vi "Final GUI.vi"() -> ()   [LabVIEW 2012]
uses:
  <vilib>/Utility/inputDevices.llb/closeJoystick.vi
  <vilib>/Utility/inputDevices.llb/joystickAcquire.vi
panel:
  in  "Request Barometer":bool
  in  "LEDs":bool
  in  "Request temperature":bool
  out "Water in control box?":bool
  out "joystick info":T1(array[cluster])
  out "Temperature (°C)":string
  out "Water Depth (cm)":string
  out "Volt (V)":string
  out "Concatenated string":string
  in  "Joystick index":i32
  in  "Local Port":u16
  out "direction info":T2
  out "button info":T3
  out "axis info":T4
  out "All Data recieved":string
  in  "Remote Port":u16
  in  "Remote Host":string
  in  "stop":bool
  # "All Data"
  # "Setup"
  # "Useless info"
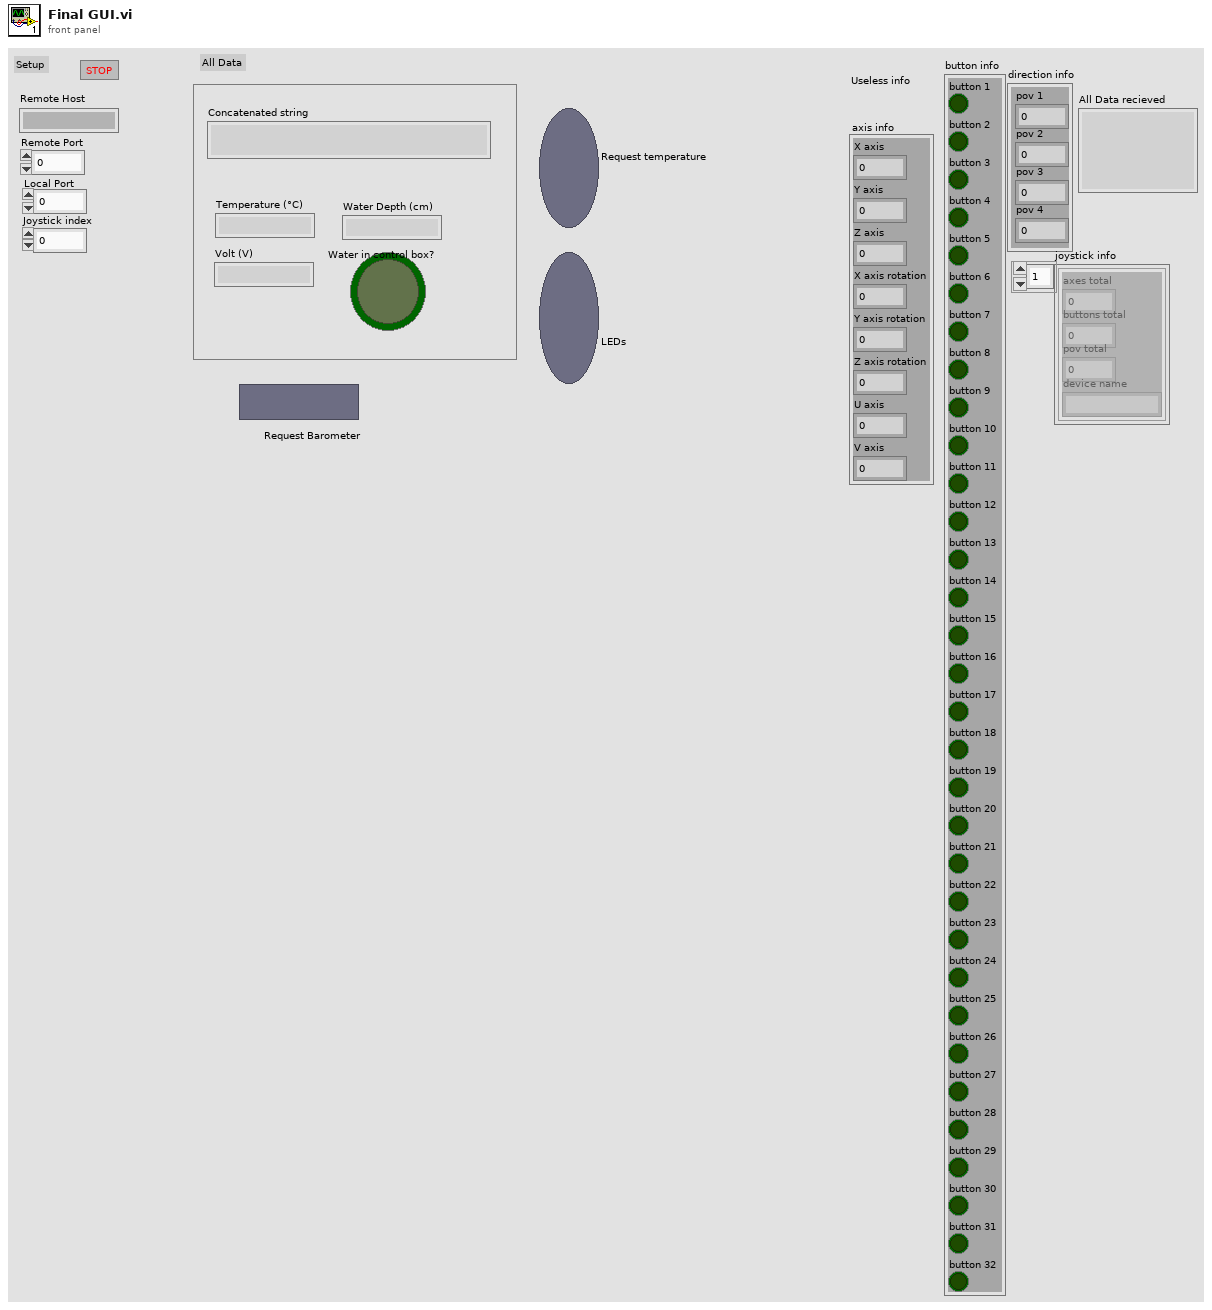
[diagram p1: front panel]
types:
  T1 = cluster{"axes total":u32, "buttons total":u32, "pov total":u32, "device name":string}[]
  T2 = cluster{"pov 1":i32, "pov 2":i32, "pov 3":i32, "pov 4":i32}
  T3 = cluster{"button 1":bool, "button 2":bool, "button 3":bool, "button 4":bool, "button 5":bool, "button 6":bool, "button 7":bool, "button 8":bool, "button 9":bool, "button 10":bool, "button 11":bool, "button 12":bool, "button 13":bool, "button 14":bool, "button 15":bool, "button 16":bool, "button 17":bool, "button 18":bool, "button 19":bool, "button 20":bool, "button 21":bool, "button 22":bool, "button 23":bool, "button 24":bool, "button 25":bool, "button 26":bool, "button 27":bool, "button 28":bool, "button 29":bool, "button 30":bool, "button 31":bool, "button 32":bool}
  T4 = cluster{"X axis":i32, "Y axis":i32, "Z axis":i32, "X axis rotation":i32, "Y axis rotation":i32, "Z axis rotation":i32, "U axis":i32, "V axis":i32}
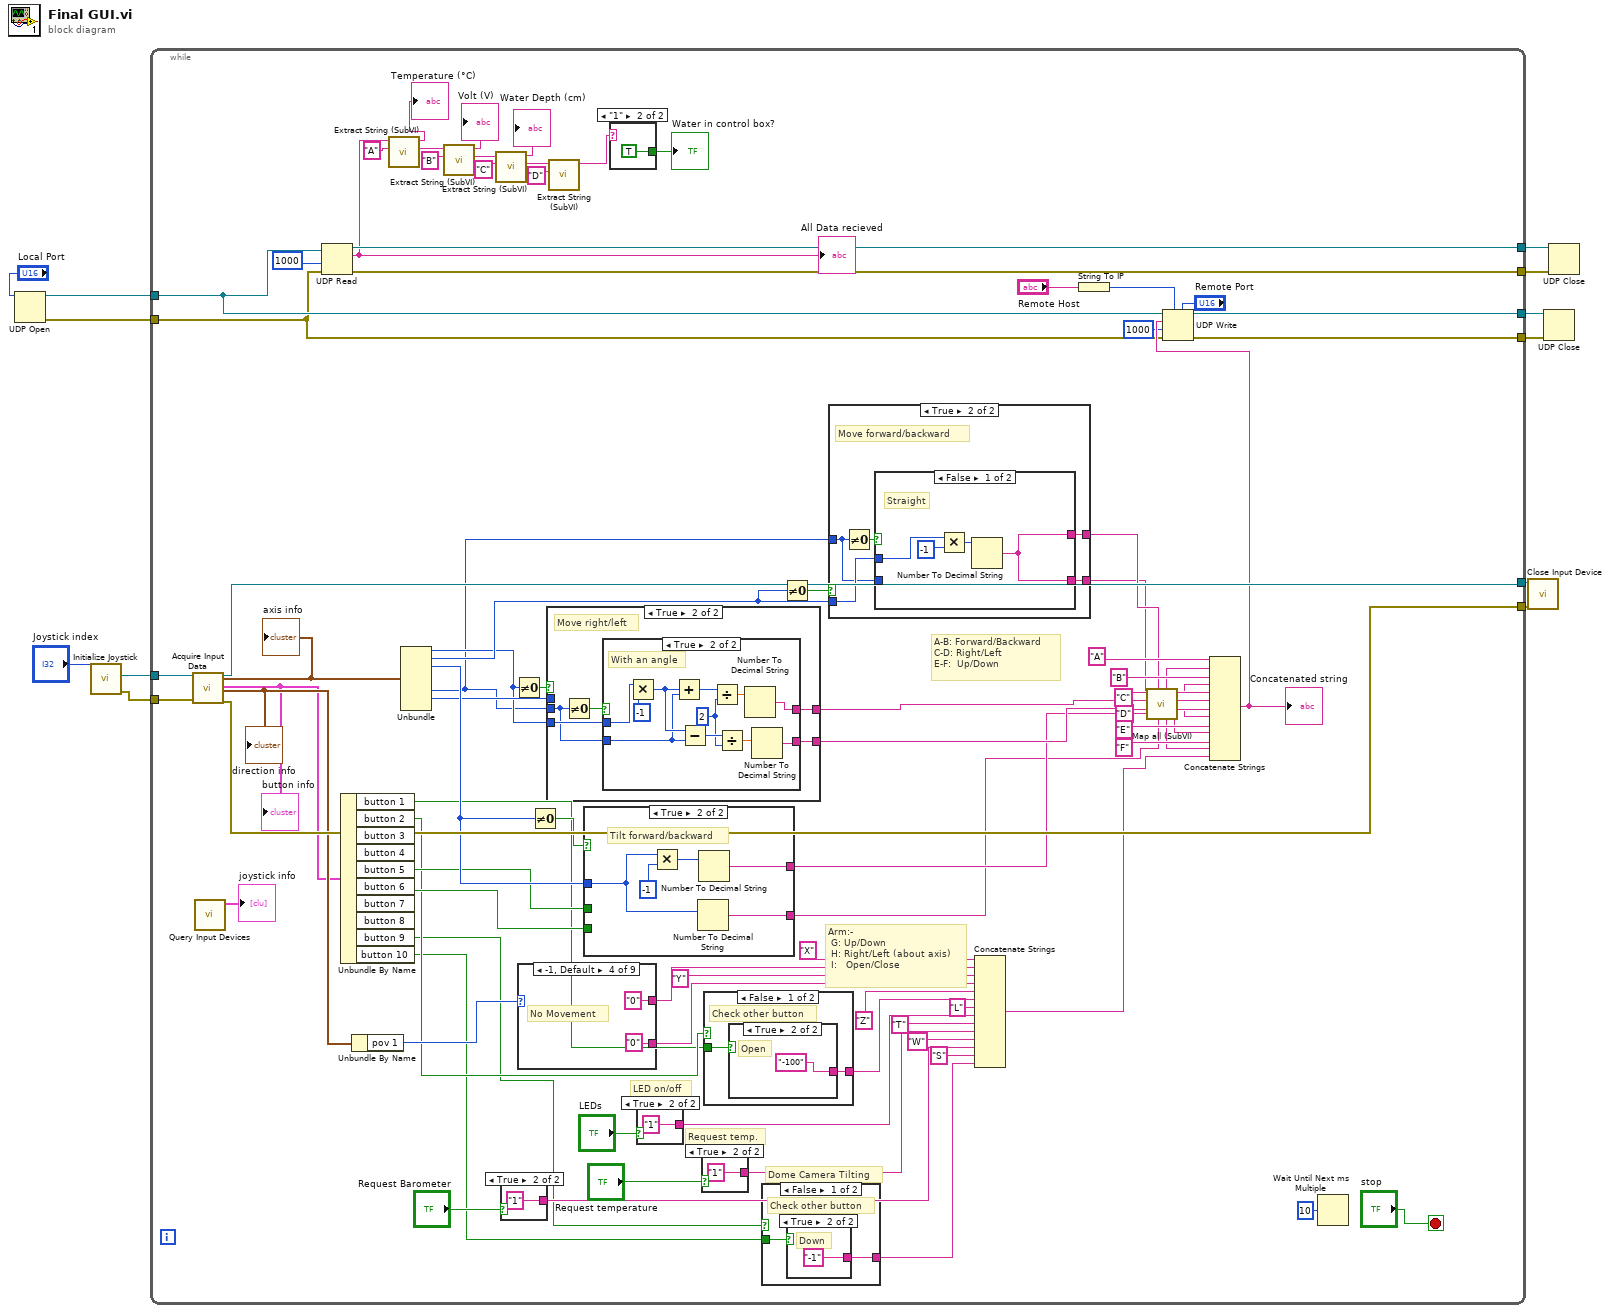
[diagram p0: block diagram]
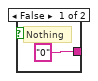
[diagram p2: hidden frame]
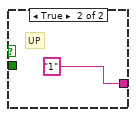
[diagram p3: hidden frame]
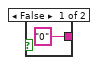
[diagram p4: hidden frame]
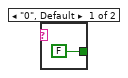
[diagram p5: hidden frame]
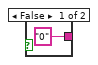
[diagram p6: hidden frame]
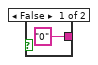
[diagram p7: hidden frame]
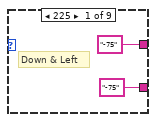
[diagram p8: hidden frame]
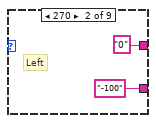
[diagram p9: hidden frame]
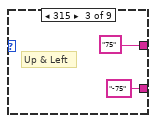
[diagram p10: hidden frame]
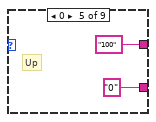
[diagram p11: hidden frame]
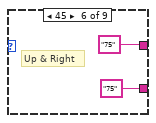
[diagram p12: hidden frame]
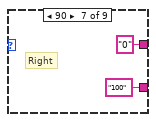
[diagram p13: hidden frame]
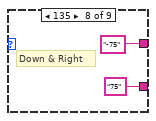
[diagram p14: hidden frame]
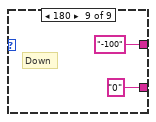
[diagram p15: hidden frame]
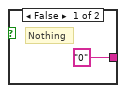
[diagram p16: hidden frame]
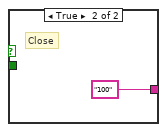
[diagram p17: hidden frame]
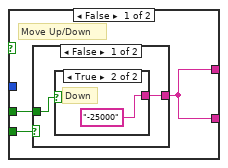
[diagram p18: hidden frame]
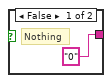
[diagram p19: hidden frame]
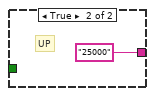
[diagram p20: hidden frame]
diagram:
  n1 = UDP Open(11:"Local Port") -> (port=w6:refnum<k16>, 0:w5:errorcluster)  [unwired: 4 in, 1 out]
  n2 = call <vilib>:"Initialize Joystick.vi"("device index"="Joystick index") -> ("error out"=w10:errorcluster, "device ID"=w11:refnum<k1>)  [unwired: 9 in]
  n3 = while {
    tunnel: w6 -> [w43]
    tunnel: w5 -> [w42]
    tunnel: w11 -> [w95]
    tunnel: w10 -> [w94]
    tunnel: [w93] -> w4
    tunnel: [w92] -> w3
    tunnel: [w91] -> w2
    tunnel: [w90] -> w1
    tunnel: [w89] -> w9
    tunnel: [w88] -> w8
    stop <- "stop" stop-if-true
    # "Dome Camera Tilting"
    # "Request temp."
    # "LED on/off"
    # "Arm:-\n G: Up/Down\n H: Right/Left (about axis)\n I:   Open/Close"
    # "A-B: Forward/Backward\nC-D: Right/Left\nE-F:  Up/Down"
    n4 = call-poly <vilib>:"Acquire Input Data.vi"("device ID"=w95, "error in (no error)"=w94) -> ("device ID"=w89:refnum<k1>, "axis info"=w97:T4, "button info"=w73:T3, "direction info"=w77:T2, "error out"=w88:errorcluster)  [unwired: 13 in]
    "axis info" <- w97
    "button info" <- w73
    "direction info" <- w77
    n5 = call <vilib>:"Query Input Devices.vi"() -> ("joystick info"=→"joystick info":T1)  [unwired: 8 in, 3 out]
    n6 = UDP Read(connection ID=w43, timeout ms (25000)=1000, 8:w42) -> (data out=w63:string, error out=w92:errorcluster, 3:w93:refnum<k16>)  [unwired: 1 in, 2 out]
    "All Data recieved" <- w63
    n7 = Unbundle By Name(w73) -> ("button 1"=w18:bool, "button 2"=w19:bool, "button 5"=w72:bool, "button 6"=w71:bool, "button 9"=w17:bool, "button 10"=w15:bool)  [unwired: 4 out]
    n8 = Unbundle By Name(w77) -> ("pov 1"=w68:i32)
    n9 = call "Extract String (SubVI).vi"("Search char"="A" ("search string/char (-)"), "Input string"=w63) -> ("Rest of text"=w61:string, "Text Extracted"=→"Temperature (°C)":string)  [unwired: 8 in]
    n10 = Unbundle(w97) -> ("X axis"=w69:i32, "Y axis"=w85:i32, "Z axis"=w74:i32, "Z axis rotation"=w53:i32, "U axis"=w70:i32)  [unwired: 3 out]
    n11 = call "Extract String (SubVI).vi"("Search char"="B" ("search string/char (-)"), "Input string"=w61) -> ("Rest of text"=w58:string, "Text Extracted"=→"Volt (V)":string)  [unwired: 8 in]
    n12 = call "Extract String (SubVI).vi"("Search char"="C" ("search string/char (-)"), "Input string"=w58) -> ("Rest of text"=w55:string, "Text Extracted"=→"Water Depth (cm)":string)  [unwired: 8 in]
    n13 = case shown="True" "Request Barometer" {
      tunnel: ["0" "1"] -> w22
      frame False {
      }
      frame True {
      }
    }
    n14 = Not Equal To 0?(x=w69) -> (x != 0?=w79:bool)
    n15 = case shown="-1, Default" w68 {
      tunnel: ["-75" "-100" "-75" "0" "0" "75" "100" "75" "0"] -> w50
      tunnel: ["-75" "0" "75" "0" "100" "75" "0" "-75" "-100"] -> w47
      frame 225 {
        # "Down & Left"
      }
      frame 270 {
        # "Left"
      }
      frame 315 {
        # "Up & Left"
      }
      frame -1, Default {
        # "No Movement"
      }
      frame 0 {
        # "Up"
      }
      frame 45 {
        # "Up & Right"
      }
      frame 90 {
        # "Right"
      }
      frame 135 {
        # "Down & Right"
      }
      frame 180 {
        # "Down"
      }
    }
    n16 = Not Equal To 0?(x=w74) -> (x != 0?=w78:bool)
    n17 = case shown="True" w79 {
      tunnel: [w151 w156] -> w36
      tunnel: w69 -> [_ w157]
      tunnel: [w152 w155] -> w35
      tunnel: w70 -> [w148 _]
      tunnel: w53 -> [_ w153]
      frame False {
        # "Tilt right/left"
        n18 = Multiply(x=w148, y=-1) -> (x*y=w149:i32)
        n19 = Number To Decimal String(number=w149) -> (decimal integer string=w151:string)  [unwired: 1 in]
        n20 = Number To Decimal String(number=w148) -> (decimal integer string=w152:string)  [unwired: 1 in]
      }
      frame True {
        # "Move right/left"
        n21 = Not Equal To 0?(x=w153) -> (x != 0?=w154:bool)
        n22 = case shown="True" w154 {
          tunnel: w157 -> [w159 w164]
          tunnel: [w158 w163] -> w156
          tunnel: [w158 w162] -> w155
          tunnel: w153 -> [_ w165]
          frame False {
            # "Normal"
            n23 = Multiply(x=-1, y=w159) -> (x*y=w161:i32)
            n24 = Number To Decimal String(number=w161) -> (decimal integer string=w158:string)  [unwired: 1 in]
          }
          frame True {
            w166 = 2 ("y")
            # "With an angle"
            n25 = Multiply(x=w164, y=-1) -> (x*y=w167:i32)
            n26 = Add(x=w167, y=w165) -> (x+y=w171:i32)
            n27 = Subtract(x=w167, y=w165) -> (x-y=w168:i32)
            n28 = Divide(x=w171, y=w166) -> (x/y=w170:dbl)
            n29 = Divide(x=w168, y=w166) -> (x/y=w169:dbl)
            n30 = Number To Decimal String(number=w170) -> (decimal integer string=w163:string)  [unwired: 1 in]
            n31 = Number To Decimal String(number=w169) -> (decimal integer string=w162:string)  [unwired: 1 in]
          }
        }
      }
    }
    n32 = call "Extract String (SubVI).vi"("Search char"="D" ("search string/char (-)"), "Input string"=w55) -> ("Text Extracted"=w20:string)  [unwired: 8 in, 1 out]
    n33 = case shown="True" w78 {
      tunnel: [w137 w143] -> w33
      tunnel: [w137 w144] -> w34
      tunnel: w74 -> [_ w145]
      tunnel: w71 -> [w136 _]
      tunnel: w72 -> [w135 _]
      frame False {
        # "Move Up/Down"
        n34 = case shown="False" w136 {
          tunnel: [w138 "25000"] -> w137
          tunnel: w135 -> [w139 _]
          frame False {
            n35 = case shown="True" w139 {
              tunnel: ["0" "-25000"] -> w138
              frame False {
                # "Nothing"
              }
              frame True {
                # "Down"
              }
            }
          }
          frame True {
            # "UP"
          }
        }
      }
      frame True {
        # "Tilt forward/backward"
        n36 = Multiply(x=w145, y=-1) -> (x*y=w147:i32)
        n37 = Number To Decimal String(number=w145) -> (decimal integer string=w143:string)  [unwired: 1 in]
        n38 = Number To Decimal String(number=w147) -> (decimal integer string=w144:string)  [unwired: 1 in]
      }
    }
    n39 = case shown="\"1\"" w20 {
      tunnel: [FALSE TRUE] -> w41
      frame "0", Default {
      }
      frame "1" {
      }
    }
    "Water in control box?" <- w41
    n40 = case shown="True" "LEDs" {
      tunnel: ["0" "1"] -> w45
      frame False {
      }
      frame True {
      }
    }
    n41 = case shown="True" "Request temperature" {
      tunnel: ["0" "1"] -> w16
      frame False {
      }
      frame True {
      }
    }
    n42 = case shown="False" w19 {
      tunnel: [w131 "100"] -> w48
      tunnel: w18 -> [w130 _]
      frame False {
        # "Check other button"
        n43 = case shown="True" w130 {
          tunnel: ["0" "-100"] -> w131
          frame False {
            # "Nothing"
          }
          frame True {
            # "Open"
          }
        }
      }
      frame True {
        # "Close"
      }
    }
    n44 = case shown="False" w17 {
      tunnel: [w100 "1"] -> w13
      tunnel: w15 -> [w99 _]
      frame False {
        # "Check other button"
        n45 = case shown="True" w99 {
          tunnel: ["0" "-1"] -> w100
          frame False {
            # "Nothing"
          }
          frame True {
            # "Down"
          }
        }
      }
      frame True {
        # "UP"
      }
    }
    n46 = Not Equal To 0?(x=w85) -> (x != 0?=w86:bool)
    n47 = case shown="True" w86 {
      tunnel: [w177 w179] -> w38
      tunnel: w85 -> [_ w181]
      tunnel: [w176 w178] -> w37
      tunnel: w53 -> [w175 w180]
      frame False {
        # "Turn right/left"
        n48 = Multiply(x=w175, y=-1) -> (x*y=w174:i32)
        n49 = Number To Decimal String(number=w175) -> (decimal integer string=w177:string)  [unwired: 1 in]
        n50 = Number To Decimal String(number=w174) -> (decimal integer string=w176:string)  [unwired: 1 in]
      }
      frame True {
        # "Move forward/backward"
        n51 = Not Equal To 0?(x=w180) -> (x != 0?=w182:bool)
        n52 = case shown="False" w182 {
          tunnel: [w183 w195] -> w179
          tunnel: w181 -> [w184 w191]
          tunnel: w180 -> [_ w190]
          tunnel: [w183 w192] -> w178
          frame False {
            # "Straight"
            n53 = Multiply(x=w184, y=-1) -> (x*y=w186:i32)
            n54 = Number To Decimal String(number=w186) -> (decimal integer string=w183:string)  [unwired: 1 in]
          }
          frame True {
            w187 = 2 ("y")
            # "With an angle"
            n55 = Multiply(x=w191, y=-1) -> (x*y=w188:i32)
            n56 = Add(x=w188, y=w190) -> (x+y=w196:i32)
            n57 = Subtract(x=w188, y=w190) -> (x-y=w189:i32)
            n58 = Divide(x=w196, y=w187) -> (x/y=w194:dbl)
            n59 = Divide(x=w189, y=w187) -> (x/y=w193:dbl)
            n60 = Number To Decimal String(number=w194) -> (decimal integer string=w195:string)  [unwired: 1 in]
            n61 = Number To Decimal String(number=w193) -> (decimal integer string=w192:string)  [unwired: 1 in]
          }
        }
      }
    }
    n62 = Concatenate Strings("X" ("string"), w47, "Y" ("string"), w50, "Z" ("string"), w48, "L" ("string"), w45, "T" ("string"), w16, "W" ("string"), w22, "S" ("string"), w13) -> (w67:string)
    n63 = String To IP(1:"Remote Host") -> (0:w65:u32)
    n64 = call "Map all (SubVI).vi"("Motor F"=w33, "Motor A"=w38, "Motor E"=w34, "Motor D"=w35, "Motor C"=w36, "Motor B"=w37) -> ("Scaled E"=w28:string, "Scaled D"=w29:string, "Scaled C"=w30:string, "Scaled B"=w31:string, "Scaled F"=w27:string, "Scaled A"=w32:string)
    n65 = Concatenate Strings("A" ("string"), w32, "B", w31, "C" ("string"), w30, "D" ("string"), w29, "E" ("string"), w28, "F" ("string"), w27, w67) -> (w76:string)
    "Concatenated string" <- w76
    n66 = UDP Write(address=w65, port or service name="Remote Port", connection ID=w43, data in=w76, 8:w42, 9:1000 ("timeout ms (25000)")) -> (error out=w90:errorcluster, 3:w91:refnum<k16>)
    n67 = Wait Until Next ms Multiple(millisecond multiple=u32 10) -> ()  [unwired: 1 out]
  }
  n68 = call-poly <vilib>:"Close Input Device.vi"("error in (no error)"=w8, "device ID"=w9) -> ()  [unwired: 8 in, 1 out]
  n69 = UDP Close(connection ID=w2, 8:w1) -> ()  [unwired: 2 out]
  n70 = UDP Close(connection ID=w4, 8:w3) -> ()  [unwired: 2 out]
